vi "Configure Temperature.vi"(0 "VISA resource name":refnum<visa-resource-name>, 5 "Thermocouple Type (0: J Type)":i32(ring) items=["J Type", "K Type", "T Type"], 7 "Temperature Unit (0: C)":i32(ring) items=["C", "F"], 9 "Simulation Value (23.00)":dbl=23.0 min=0.0 max=50.0 step=0.01 format="%#.2f", 11 "error in (no error)":errorcluster) -> (4 "VISA resource name out":refnum<visa-resource-name>, 15 "error out":errorcluster)   [LabVIEW 2021, in "GWInstek  GDM8351.lvlib"]
doc: "Configures the thermocouple type, unit, simulation value for temperature."
uses:
  <instrlib>/GWInstek  GDM8351/GWInstek  GDM8351.lvlib
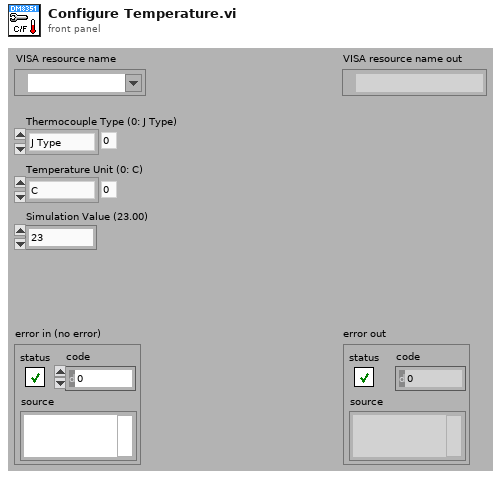
[diagram p1: front panel]
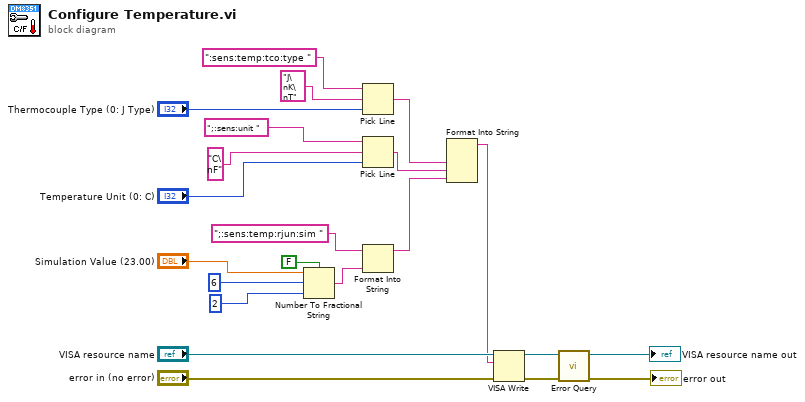
[diagram p0: block diagram]
diagram:
  n1 = Number To Fractional String(use system decimal point (T)=FALSE, number="Simulation Value (23.00)", width (-)=i16 6, precision (6)=i16 2) -> (F-format string=w15:string)
  n2 = Pick Line(string ("")=":sens:temp:tco:type ", multi-line string="J\nK\nT", line index="Thermocouple Type (0: J Type)") -> (output string=w5:string)
  n3 = Pick Line(string ("")=";:sens:unit ", multi-line string="C\nF", line index="Temperature Unit (0: C)") -> (output string=w6:string)
  n4 = Format Into String(initial string=";:sens:temp:rjun:sim ", w15) -> (resulting string=w2:string)  [unwired: 2 in, 1 out]
  n5 = Format Into String(w5, w6, w2) -> (resulting string=w4:string)  [unwired: 3 in, 1 out]
  n6 = VISA Write(VISA resource name="VISA resource name", write buffer=w4, error in (no error)="error in (no error)") -> (VISA resource name out=w11:refnum<visa-resource-name>, error out=w10:errorcluster)  [unwired: 1 out]
  n7 = call <instrlib>:"Error Query.vi"("error in (no error)"=w10, "VISA resource name"=w11) -> ("error out"=→"error out":errorcluster, "VISA resource name out"=→"VISA resource name out":refnum<visa-resource-name>)  [unwired: 6 in, 2 out]
